vi "Configure Feed Forward Equalization Characteristics.vi"(5 "Vertical Range (64)":dbl=64.0, 6 "Vertical Offset (0 Volt)":dbl, 7 "Scale Type (1: Manual)":i32(ring)=1 items=["Auto", "Manual"], 8 "error in (no error)":errorcluster, 9 "Data Rate (1E+9)":dbl=1000000000.0, 10 "Precursor Taps (0)":dbl, 11 "VISA resource name":refnum<visa-resource-name>) -> (0 "error out":errorcluster, 3 "VISA resource name out":refnum<visa-resource-name>)   [LabVIEW 2013, in "Agilent 90000 Series.lvlib"]
doc: "Configures advance settings for Feed Forward Equalization."
uses:
  Agilent 90000 Series.lvlib
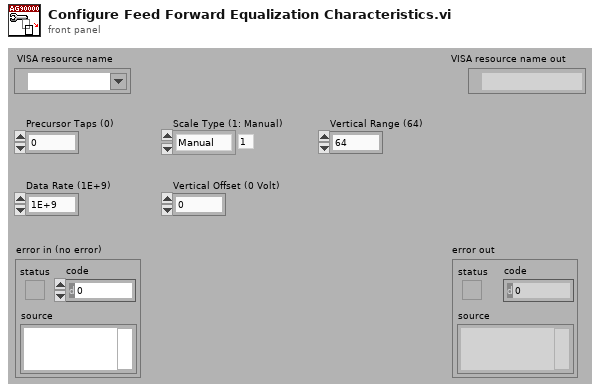
[diagram p1: front panel]
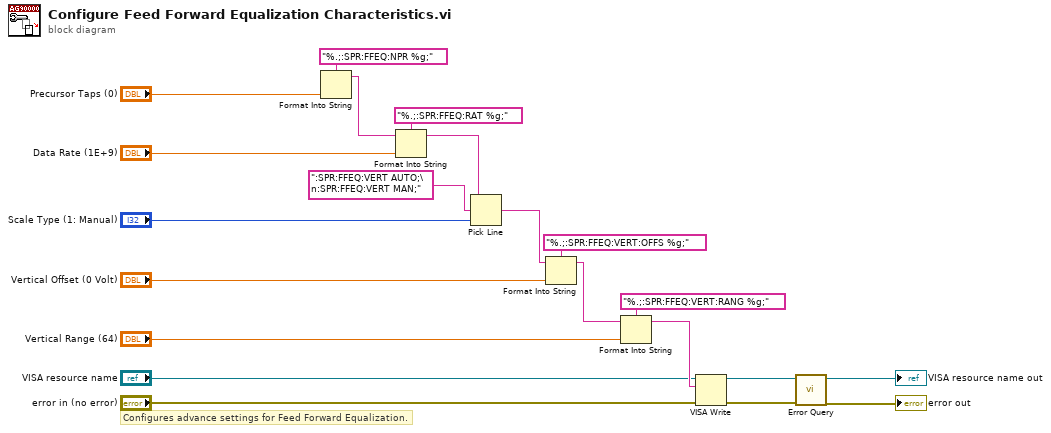
[diagram p0: block diagram]
diagram:
  # "Configures advance settings for Feed Forward Equalization."
  n1 = Format Into String(format string="%.;:SPR:FFEQ:NPR %g;", "Precursor Taps (0)") -> (resulting string=w19:string)  [unwired: 2 in, 1 out]
  n2 = Format Into String(format string="%.;:SPR:FFEQ:RAT %g;", initial string=w19, "Data Rate (1E+9)") -> (resulting string=w14:string)  [unwired: 1 in, 1 out]
  n3 = Pick Line(string ("")=w14, multi-line string=":SPR:FFEQ:VERT AUTO;\n:SPR:FFEQ:VERT MAN;", line index="Scale Type (1: Manual)") -> (output string=w13:string)
  n4 = Format Into String(format string="%.;:SPR:FFEQ:VERT:OFFS %g;", initial string=w13, "Vertical Offset (0 Volt)") -> (resulting string=w10:string)  [unwired: 1 in, 1 out]
  n5 = Format Into String(format string="%.;:SPR:FFEQ:VERT:RANG %g;", initial string=w10, "Vertical Range (64)") -> (resulting string=w7:string)  [unwired: 1 in, 1 out]
  n6 = VISA Write(VISA resource name="VISA resource name", write buffer=w7, error in (no error)="error in (no error)") -> (VISA resource name out=w4:refnum<visa-resource-name>, error out=w3:errorcluster)  [unwired: 1 out]
  n7 = call "Error Query.vi"("error in (no error)"=w3, "VISA resource name"=w4) -> ("error out"=→"error out":errorcluster, "VISA resource name out"=→"VISA resource name out":refnum<visa-resource-name>)  [unwired: 8 out]
